vi "获取蓄电池信息.vi"(8 "error in (no error)":errorcluster, 11 "MB session in":refnum<class "MB_Master.lvclass">) -> (0 "error out":errorcluster, 2 "蓄电池信息":T1, 3 "MB session out":refnum<class "MB_Master.lvclass">)   [LabVIEW 2016, in "环境动力单元.lvlib"]
uses:
  <vilib>/Plasmionique/MB Master/MB_Master/MB_Master.lvclass
  <vilib>/Plasmionique/MB Master/MB Master.lvlib
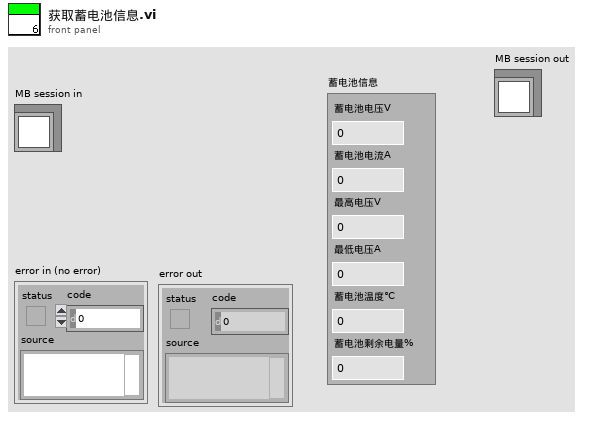
[diagram p1: front panel]
types:
  T1 = cluster{"蓄电池电压V":dbl, "蓄电池电流A":dbl, "最高电压V":dbl, "最低电压A":dbl, "蓄电池温度℃":dbl, "蓄电池剩余电量%":dbl}
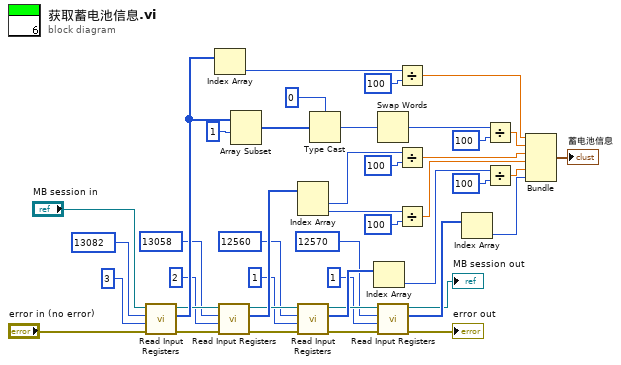
[diagram p0: block diagram]
diagram:
  n1 = call <vilib>:"Read Input Registers.vi"("error in (no error)"="error in (no error)", "quantity"=u16 3, "starting address"=u16 13082, "MB session in"="MB session in") -> ("error out"=w25:errorcluster, "Registers"=w40:u16[], "MB session out"=w27:refnum<class "MB_Master.lvclass">)  [unwired: 5 in]
  n2 = Index Array(array=w40) -> (element=w37:u16)  [unwired: 1 in]
  n3 = call <vilib>:"Read Input Registers.vi"("error in (no error)"=w25, "quantity"=u16 2, "starting address"=u16 13058, "MB session in"=w27) -> ("error out"=w16:errorcluster, "Registers"=w22:u16[], "MB session out"=w15:refnum<class "MB_Master.lvclass">)  [unwired: 5 in]
  n4 = Array Subset(array=w40, index=1 ("索引")) -> (w33:u16[])  [unwired: 1 in]
  n5 = Index Array(array=w22) -> (element #1=w21:u16, element #2=w19:u16)  [unwired: 2 in]
  n6 = call <vilib>:"Read Input Registers.vi"("error in (no error)"=w16, "quantity"=u16 1, "starting address"=u16 12560, "MB session in"=w15) -> ("error out"=w9:errorcluster, "Registers"=w13:u16[], "MB session out"=w7:refnum<class "MB_Master.lvclass">)  [unwired: 5 in]
  n7 = Type Cast(type=0, x=w33) -> (*(type *) &x=w31:i32)
  n8 = Index Array(array=w13) -> (element=w11:u16)  [unwired: 1 in]
  n9 = Swap Words(1:w31) -> (0:w30:i32)
  n10 = call <vilib>:"Read Input Registers.vi"("error in (no error)"=w9, "quantity"=u16 1, "starting address"=u16 12570, "MB session in"=w7) -> ("error out"=→"error out":errorcluster, "Registers"=w3:u16[], "MB session out"=→"MB session out":refnum<class "MB_Master.lvclass">)  [unwired: 5 in]
  n11 = Divide(x=w37, y=u16 100) -> (x/y=w35:dbl)
  n12 = Divide(x=w21, y=100) -> (x/y=w18:dbl)
  n13 = Divide(x=w19, y=100) -> (x/y=w17:dbl)
  n14 = Index Array(array=w3) -> (element=w2:u16)  [unwired: 1 in]
  n15 = Divide(x=w30, y=100) -> (x/y=w28:dbl)
  n16 = Divide(x=w11, y=100) -> (x/y=w10:dbl)
  n17 = Bundle(w35, w28, w18, w17, w10, w2) -> (→"蓄电池信息":cluster{dbl, dbl, dbl, dbl, dbl, u16})  [unwired: 1 in]
